vi "Max_Min_Limiter.vi"(2 "Analysis info":T2={"Colour"=0, "Inst type"=enum."Pitot-static tube", "Inst name"="Manometer voltage", "Symbol"="U", "Code name"="", "Extra Info"="U", "Inst Array"=enum."PWA", "U"=0.0, "u^2"=0.0, "u^3"=0.0, "u^4"=0.0, "Skew_u"=0.0, "Kurt_u"=0.0, "Sd Error in Mean"=0.0, "% u'/U"=0.0, "X"=0.0, "Y"=0.0, "Z"=0.0, "Timescale integral Estimate"=0.0, "Sd Error in Variance"=0.0, "Calib File"=path "", "Calib Constants"=[], "Output Position"=FALSE, "Stats"=enum."None", "Av Sampling Rate"=0.0, "Av No of Samples"=0.0, "Total Meas Time (s)"=0.0, "OrigChName"="", "Max value"=0.0, "Min value"=0.0, "Req Sample Rate Hz"=0.0, "Sync Delay Time (s)"=0.0, "Ch No"=0, "Device"="", "Use Latest Calib"=FALSE, "Port"="", "Metadata Ch Names"=[], "Metadata Ch Values"=[], "Label"="", "chState"=enum."Solo", "Point Drift"=0.0, "inputConfig"=""} {"Kurt_u" format="%_3g"; "u^4" format="%_3g"; "u^3" format="%_3g"; "Sd Error in Variance" format="%_3g"; "u^2" format="%_3g"; "Sd Error in Mean" format="%_3g"; "U" format="%_3g"; "Sync Delay Time (s)" format="%.4f"; "Total Meas Time (s)" format="%_5g"; "Skew_u" format="%_3g"; "% u'/U" format="%_3g"}, 3 "Time Trace In":T1) -> (1 "Time Trace Out":T1)   [LabVIEW 2022 SP3]
uses:
  <vilib>/Analysis/NI_AALBase.lvlib
  Globals/Meas_global.vi
  Controls/Post_Process.ctl
  Controls/Inst_type.ctl
  Controls/Instrument_Array.ctl
  Controls/Analysis_info_cluster.ctl
  Controls/Time_Trace_Cluster.ctl
  Controls/channelState.ctl
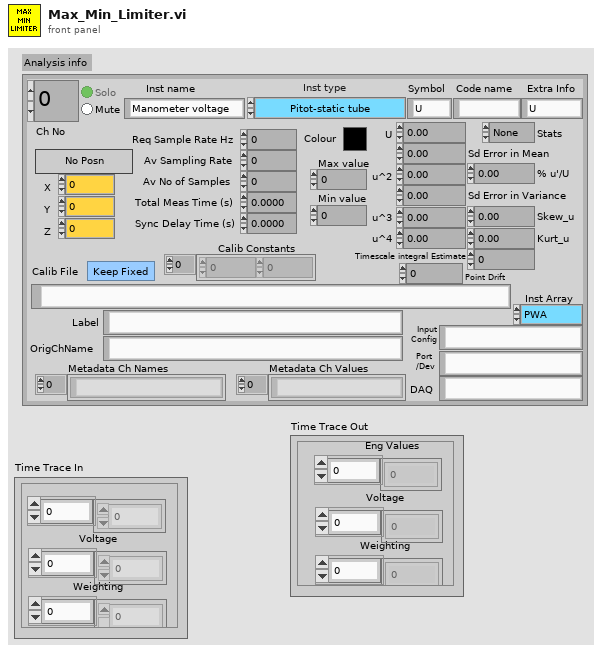
[diagram p1: front panel]
types:
  T1 = typedef "Time_Trace_Cluster.ctl" = cluster{"Weighting":dbl[], "Voltage":dbl[], "Eng Values":dbl[]}
  T2 = typedef "Analysis_info_cluster.ctl" = cluster{"Colour":u32, "Inst type":T3, "Inst name":string, "Symbol":string, "Code name":string, "Extra Info":string, "Inst Array":T4, "U":dbl, "u^2":dbl, "u^3":dbl, "u^4":dbl, "Skew_u":dbl, "Kurt_u":dbl, "Sd Error in Mean":dbl, "% u'/U":dbl, "X":dbl, "Y":dbl, "Z":dbl, "Timescale integral Estimate":dbl, "Sd Error in Variance":dbl, "Calib File":path, "Calib Constants":dbl[], "Output Position":bool, "Stats":enum16{"None", "Basic", "Full"}, "Av Sampling Rate":dbl, "Av No of Samples":dbl, "Total Meas Time (s)":dbl, "OrigChName":string, "Max value":dbl, "Min value":dbl, "Req Sample Rate Hz":dbl, "Sync Delay Time (s)":dbl, "Ch No":i16, "Device":string, "Use Latest Calib":bool, "Port":string, "Metadata Ch Names":string[], "Metadata Ch Values":string[], "Label":string, "chState":T5, "Point Drift":dbl, "inputConfig":string}
  T3 = typedef "Inst_type.ctl" = enum16{"Raw voltage", "Raw with zero offsetting", "Propeller anemometer", "Pressure Transducer", "Pitot-static tube", "Hot wire", "Cross wire 1", "Cross wire 2", "Generic Linear", "Generic Polynomial", "Generic BackPoly", "Fast FID", "Thermocouple", "Cold wire", "Pulsed Wire", "LDA Vel", "LDA Tran time", "LDA Arr time", "Microphone"}
  T4 = typedef "Instrument_Array.ctl" = enum16{"PWA", "LDA", "Analogue"}
  T5 = typedef "channelState.ctl" = enum32{"No Selection", "Solo", "Mute"}
  T6 = typedef "Post_Process.ctl" = enum16{"Take New Data", "Post Process Raw Data File"}
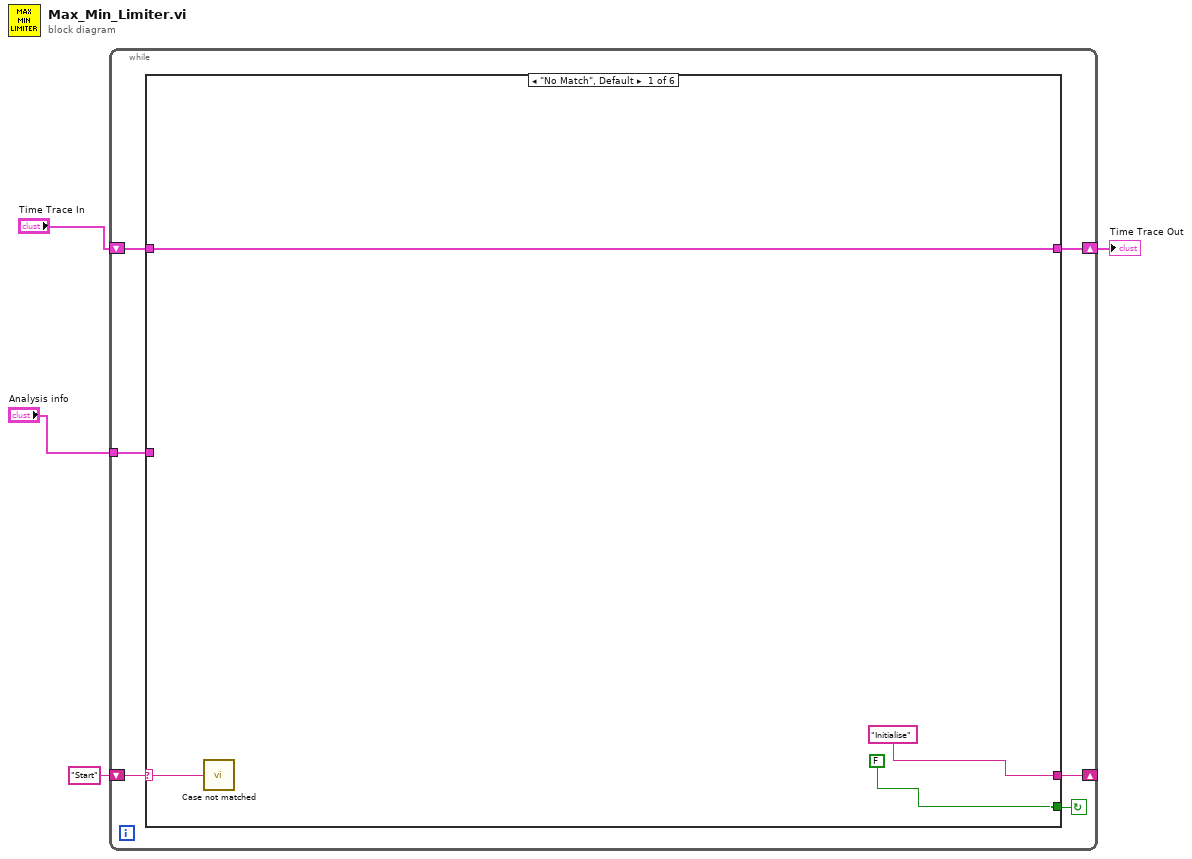
[diagram p0: block diagram]
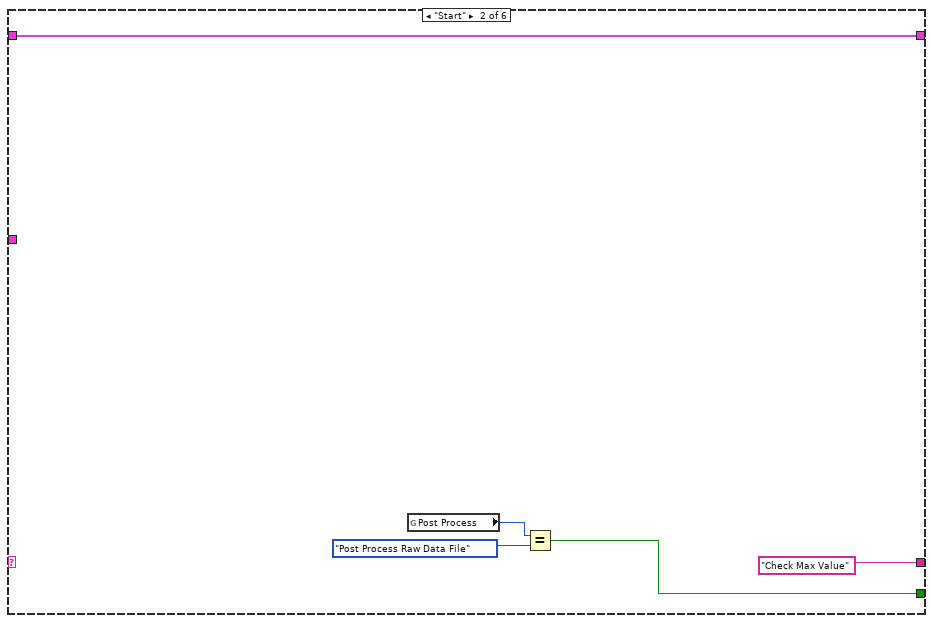
[diagram p2: hidden frame]
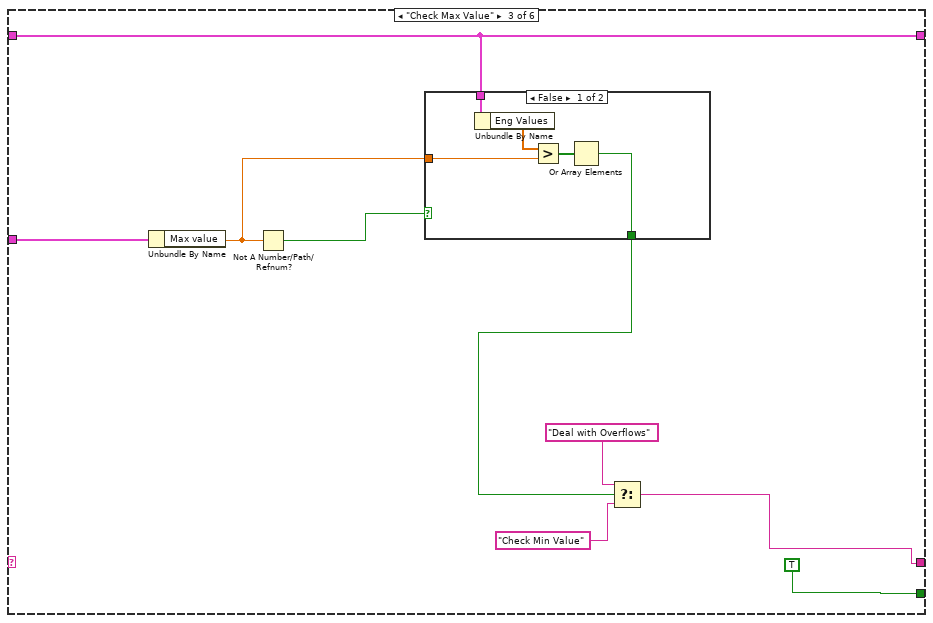
[diagram p3: hidden frame]
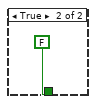
[diagram p4: hidden frame]
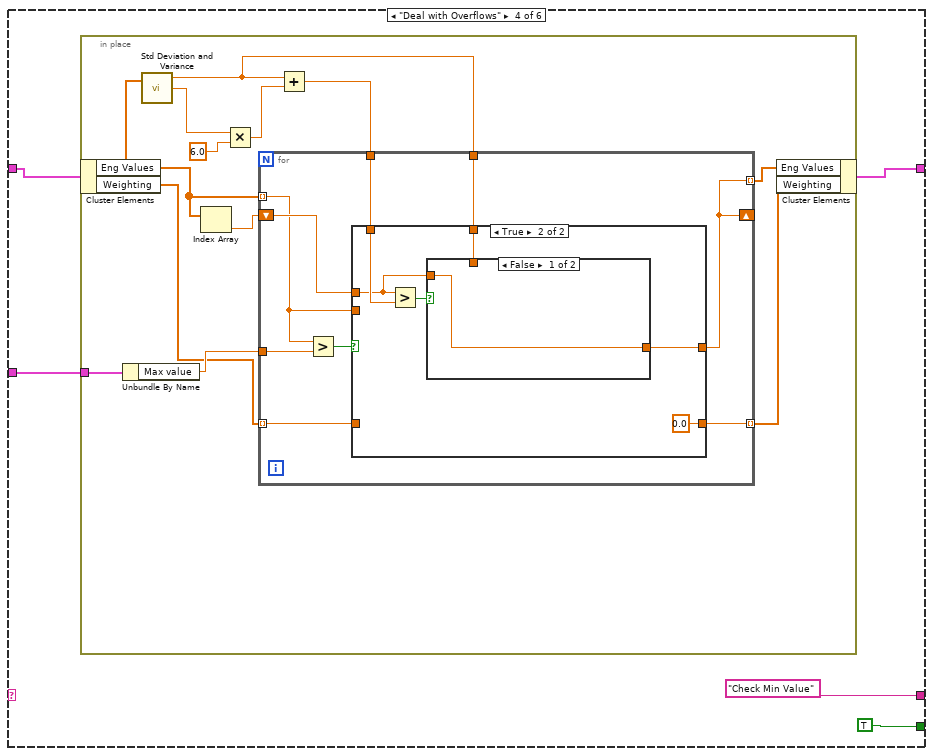
[diagram p5: hidden frame]
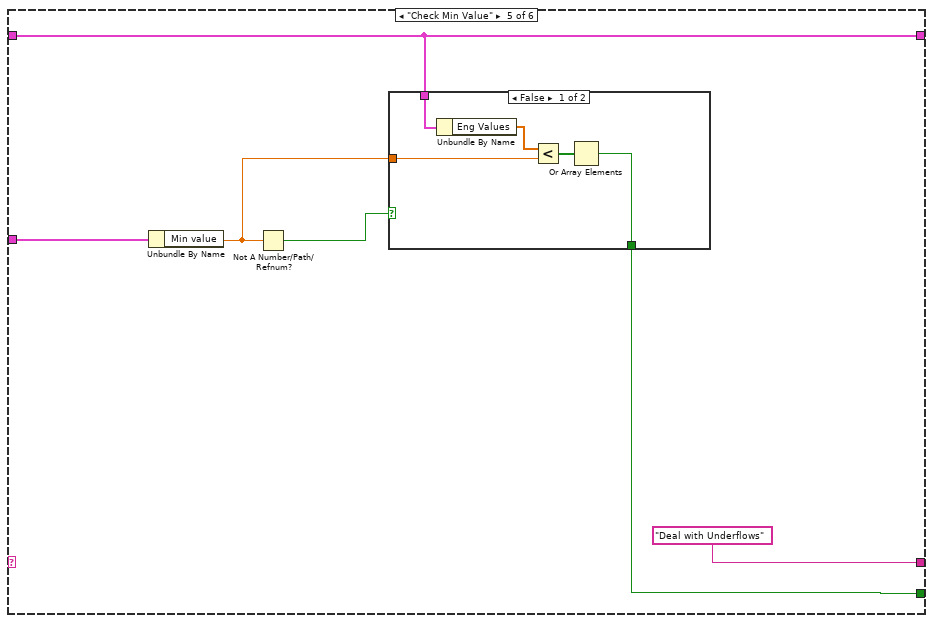
[diagram p8: hidden frame]
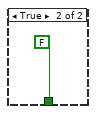
[diagram p9: hidden frame]
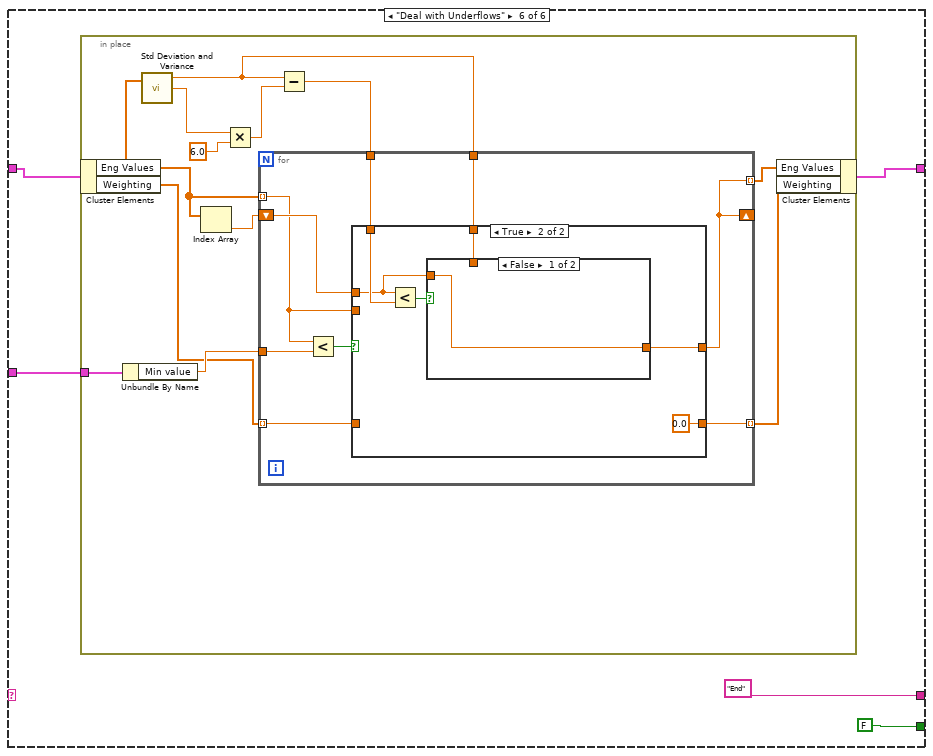
[diagram p10: hidden frame]
diagram:
  n1 = while {
    shift-left: "Start" ("f") -> [w8]
    shift-right: [w9] -> _
    tunnel: "Analysis info" -> [w7]
    shift-right: [w5] -> w2
    shift-left: "Time Trace In" -> [w6]
    stop <- w10 continue-if-true
    n2 = case shown="\"No Match\", Default" w8 {
      selector: w8 -> [w11 _ _ _ _ _]
      tunnel: [FALSE w16 TRUE TRUE w72 FALSE] -> w10
      tunnel: ["Initialise" "Check Max Value" w26 "Check Min Value" "Deal with Underflows" ("f") "End"] -> w9
      tunnel: w7 -> [_ _ w27 w37 w76 w85]
      tunnel: w6 -> [w12 w15 w20 w36 w71 w84]
      tunnel: [w12 w15 w20 w35 w71 w83] -> w5
      frame "No Match", Default {
        n3 = call "Case not matched.vi"("Case Name not Matched"=w11) -> ()
      }
      frame "Start" {
        n4 = global read "Meas_global.vi" "Post Process"() -> (w17:T6)
        n5 = Equal?(x=w17, y=Post_Process."Post Process Raw Data File" ("Post Process")) -> (x = y?=w16:bool)
      }
      frame "Check Max Value" {
        n6 = Unbundle By Name(w27) -> ("Max value"=w24:dbl)
        n7 = Not A Number/Path/Refnum?(number/path/refnum=w24) -> (NaN/Path/Refnum?=w25:bool)
        n8 = case shown="False" w25 {
          tunnel: w20 -> [w31 _]
          tunnel: w24 -> [w33 _]
          tunnel: [w32 FALSE] -> w23
          frame False {
            n9 = Unbundle By Name(w31) -> ("Eng Values"=w30:dbl[])
            n10 = Greater?(x=w30, y=w33) -> (0:w29:bool[])
            n11 = Or Array Elements(Boolean array=w29) -> (logical OR=w32:bool)
          }
          frame True {
          }
        }
        n12 = Select(t="Deal with Overflows" ("f"), s=w23, f="Check Min Value") -> (s? t:f=w26:string)
      }
      frame "Deal with Overflows" {
        n13 = in-place {
          in-place-border: w37 -> [w51]
          n14 = in-place-cluster #1(w36) -> ("Eng Values"=w43:dbl[], "Weighting"=w42:dbl[])
          n15 = Unbundle By Name(w51) -> ("Max value"=w50:dbl)
          n16 = call <vilib>:"Std Deviation and Variance.vi"("X"=w43) -> ("mean"=w44:dbl, "standard deviation"=w48:dbl)  [unwired: 1 in, 1 out]
          n17 = Index Array(array=w43) -> (element=w49:dbl)  [unwired: 1 in]
          n18 = Multiply(x=w48, y=6.0) -> (x*y=w46:dbl)
          n19 = Add(x=w44, y=w46) -> (x+y=w45:dbl)
          n20 = for {
            tunnel: w43 -> [w55] mode=indexing
            tunnel: w50 -> [w60]
            shift-right: [w54] -> _
            shift-left: w49 -> [w58]
            tunnel: w45 -> [w57]
            tunnel: w44 -> [w56]
            tunnel: [w54] -> w41 mode=indexing
            tunnel: [w53] -> w40 mode=indexing
            tunnel: w42 -> [w52] mode=indexing
            n21 = Greater?(x=w55, y=w60) -> (0:w59:bool)
            n22 = case shown="True" w59 {
              tunnel: w58 -> [_ w64]
              tunnel: w57 -> [_ w68]
              tunnel: [w62 w66] -> w54
              tunnel: w56 -> [_ w65]
              tunnel: w55 -> [w62 _]
              tunnel: [w61 0.0 ("Numeric")] -> w53
              tunnel: w52 -> [w61 _]
              frame False {
              }
              frame True {
                n23 = Greater?(x=w64, y=w68) -> (0:w67:bool)
                n24 = case shown="False" w67 {
                  tunnel: [w69 w70] -> w66
                  tunnel: w65 -> [_ w70]
                  tunnel: w64 -> [w69 _]
                  frame False {
                  }
                  frame True {
                  }
                }
              }
            }
          }
          n25 = in-place-cluster #1("Eng Values"=w41, "Weighting"=w40) -> (w35:T1)
        }
      }
      frame "Check Min Value" {
        n26 = Unbundle By Name(w76) -> ("Min value"=w74:dbl)
        n27 = Not A Number/Path/Refnum?(number/path/refnum=w74) -> (NaN/Path/Refnum?=w75:bool)
        n28 = case shown="False" w75 {
          tunnel: w71 -> [w79 _]
          tunnel: w74 -> [w81 _]
          tunnel: [w80 FALSE] -> w72
          frame False {
            n29 = Unbundle By Name(w79) -> ("Eng Values"=w78:dbl[])
            n30 = Less?(x=w78, y=w81) -> (x < y?=w77:bool[])
            n31 = Or Array Elements(Boolean array=w77) -> (logical OR=w80:bool)
          }
          frame True {
          }
        }
      }
      frame "Deal with Underflows" {
        n32 = in-place {
          in-place-border: w85 -> [w99]
          n33 = in-place-cluster #2(w84) -> ("Eng Values"=w91:dbl[], "Weighting"=w90:dbl[])
          n34 = Unbundle By Name(w99) -> ("Min value"=w98:dbl)
          n35 = call <vilib>:"Std Deviation and Variance.vi"("X"=w91) -> ("mean"=w92:dbl, "standard deviation"=w96:dbl)  [unwired: 1 in, 1 out]
          n36 = Index Array(array=w91) -> (element=w97:dbl)  [unwired: 1 in]
          n37 = Multiply(x=w96, y=6.0) -> (x*y=w94:dbl)
          n38 = Subtract(x=w92, y=w94) -> (x-y=w93:dbl)
          n39 = for {
            tunnel: w91 -> [w103] mode=indexing
            tunnel: w98 -> [w108]
            shift-right: [w102] -> _
            shift-left: w97 -> [w106]
            tunnel: w93 -> [w105]
            tunnel: w92 -> [w104]
            tunnel: [w102] -> w89 mode=indexing
            tunnel: [w101] -> w88 mode=indexing
            tunnel: w90 -> [w100] mode=indexing
            n40 = Less?(x=w103, y=w108) -> (x < y?=w107:bool)
            n41 = case shown="True" w107 {
              tunnel: w106 -> [_ w112]
              tunnel: w105 -> [_ w116]
              tunnel: [w110 w114] -> w102
              tunnel: w104 -> [_ w113]
              tunnel: w103 -> [w110 _]
              tunnel: [w109 0.0 ("Numeric")] -> w101
              tunnel: w100 -> [w109 _]
              frame False {
              }
              frame True {
                n42 = Less?(x=w112, y=w116) -> (x < y?=w115:bool)
                n43 = case shown="False" w115 {
                  tunnel: [w117 w118] -> w114
                  tunnel: w113 -> [_ w118]
                  tunnel: w112 -> [w117 _]
                  frame False {
                  }
                  frame True {
                  }
                }
              }
            }
          }
          n44 = in-place-cluster #2("Eng Values"=w89, "Weighting"=w88) -> (w83:T1)
        }
      }
    }
  }
  "Time Trace Out" <- w2
